vi "Shortcut Menu from Cluster.vi"() -> ()   [LabVIEW 2019]
doc: "An example of using a cluster of enums and booleans to provide menu options, both for the right-click menu of a control, and in the VI menu bar."
uses:
  vi.lib/JDP Science/JDP Science Common Utilities/Shortcut Menu Tools/Menu From Cluster.lvlib
panel:
  out "Item":string
  out "ItemTag":string
  out "A control":dbl caption="Run this program, then right-click this control and experiment changing Options"
  # "This example also shows how to add the same Options to the VI's menu bar (under \"User Options\")."
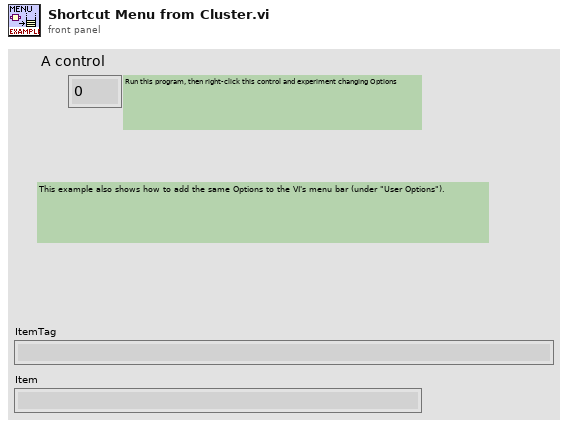
[diagram p1: front panel]
types:
  T1 = cluster{"An Enum":enum16{"Item1", "Item2", "Item3"}, "A Boolean":bool, "Another boolean":bool, "A subcluster":cluster{"Sub Enum":enum16{"Item1", "Item2", "Item3"}, "Sub Boolean":bool, "Subsubcluster":cluster{"Sub Sub Enum":enum16{"Item1", "Item2", "Item3"}, "Sub Sub Boolean":bool, "3sub":cluster{"3sub Enum":enum16{"Item1", "Item2", "Item3"}, "3sub Boolean":bool}}}}
  T2 = cluster{"Options Menu":cluster{"An Enum":enum16{"Item1", "Item2", "Item3"}, "A Boolean":bool, "Another boolean":bool, "A subcluster":cluster{"Sub Enum":enum16{"Item1", "Item2", "Item3"}, "Sub Boolean":bool, "Subsubcluster":cluster{"Sub Sub Enum":enum16{"Item1", "Item2", "Item3"}, "Sub Sub Boolean":bool, "3sub":cluster{"3sub Enum":enum16{"Item1", "Item2", "Item3"}, "3sub Boolean":bool}}}}}
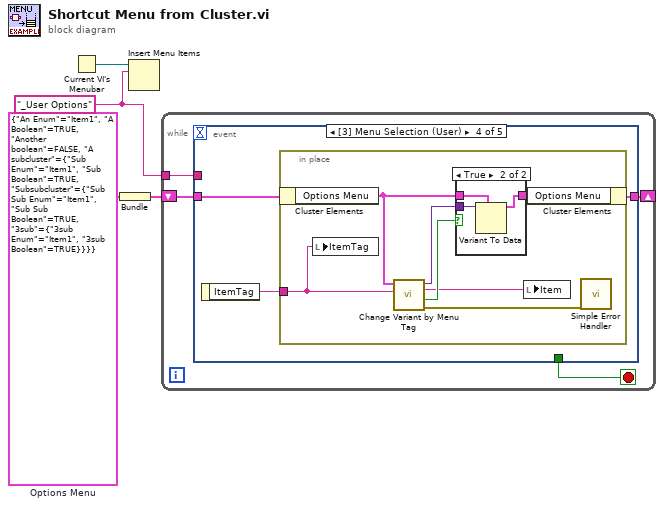
[diagram p0: block diagram]
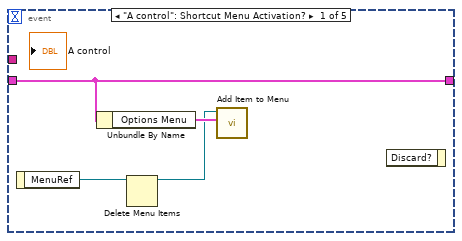
[diagram p2: hidden frame]
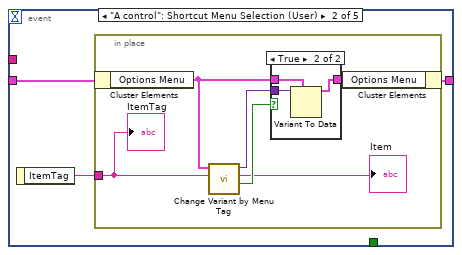
[diagram p3: hidden frame]
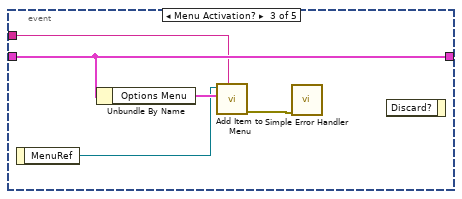
[diagram p5: hidden frame]
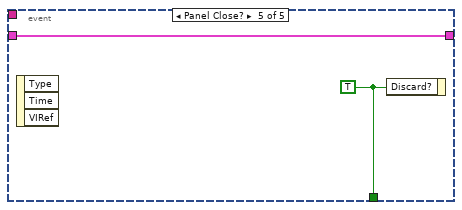
[diagram p7: hidden frame]
diagram:
  w1 = "_User Options" ("menu tag")
  w3 = T1 {"An Enum"=enum."Item1", "A Boolean"=TRUE, "Another boolean"=FALSE, "A subcluster"={"Sub Enum"=enum."Item1", "Sub Boolean"=TRUE, "Subsubcluster"={"Sub Sub Enum"=enum."Item1", "Sub Sub Boolean"=TRUE, "3sub"={"3sub Enum"=enum."Item1", "3sub Boolean"=TRUE}}}}  # Options Menu
  n1 = Current VI's Menubar() -> (w2:refnum<k9>)
  n2 = Bundle("Options Menu"=w3) -> (w4:T2)  [unwired: 1 in]
  n3 = Insert Menu Items(8:w1, 9:w2) -> ()  [unwired: 4 in, 3 out]
  n4 = while {
    shift-right: [w7] -> _
    shift-left: w4 -> [w8]
    tunnel: w1 -> [w5]
    stop <- w6 stop-if-true
    n5 = event shown="[3] Menu Selection (User)" {
      selector: _ -> [_ _ _ _ _]
      dyn-events: _ -> [_ _ _ _ _]
      timeout: _ -> [_ _ _ _ _]
      tunnel: w8 -> [w12 w15 w30 w33 w46]
      tunnel: [w12 w14 w30 w32 w46] -> w7
      tunnel: [_ _ _ _ w45] -> w6
      tunnel: w5 -> [_ _ w28 _ _]
      event "A control": Shortcut Menu Activation? {
        n6 = event-data() -> ("MenuRef"=w11:refnum<k9>)  [unwired: 1 in]
        n7 = Unbundle By Name(w12) -> ("Options Menu"=w10:T1)
        n8 = Delete Menu Items(9:w11) -> (3:w9:refnum<k9>)  [unwired: 3 in, 1 out]
        n9 = call "Add Item to Menu.vi"("Item(s) to Add"=w10, "menu reference"=w9) -> ()  [unwired: 7 in, 3 out]
        n10 = event-data() -> ()  [unwired: 2 in, 1 out]
      }
      event "A control": Shortcut Menu Selection (User) {
        n11 = event-data() -> ("ItemTag"=w13:string)  [unwired: 1 in]
        n12 = in-place {
          in-place-border: w13 -> [w17]
          n13 = in-place-cluster #1(w15) -> ("Options Menu"=w20:T1)
          n14 = call "Change Variant by Menu Tag.vi"("tag"=w17, "Cluster"=w20) -> ("Cluster Changed"=w18:bool, "Item"=→"Item":string, "VCluster out"=w19:variant)  [unwired: 6 in, 1 out]
          n15 = case shown="True" w18 {
            tunnel: w19 -> [_ w25]
            tunnel: [w22 w24] -> w21
            tunnel: w20 -> [w22 w23]
            frame False {
            }
            frame True {
              n16 = Variant To Data(type=w23, Variant=w25) -> (data=w24:T1)  [unwired: 1 in, 1 out]
            }
          }
          n17 = in-place-cluster #1("Options Menu"=w21) -> (w14:T2)
          "ItemTag" <- w17
        }
      }
      event Menu Activation? {
        n18 = event-data() -> ("MenuRef"=w27:refnum<k9>)  [unwired: 1 in]
        n19 = Unbundle By Name(w30) -> ("Options Menu"=w29:T1)
        n20 = call "Add Item to Menu.vi"("menu tag"=w28, "Item(s) to Add"=w29, "menu reference"=w27) -> ("error out"=w26:errorcluster)  [unwired: 6 in, 2 out]
        n21 = call <vilib>:"Simple Error Handler.vi"("error in (no error)"=w26) -> ()  [unwired: 4 in, 5 out]
        n22 = event-data() -> ()  [unwired: 2 in, 1 out]
      }
      event Menu Selection (User) {
        n23 = event-data() -> ("ItemTag"=w31:string)  [unwired: 1 in]
        n24 = in-place {
          in-place-border: w31 -> [w36]
          n25 = in-place-cluster #2(w33) -> ("Options Menu"=w39:T1)
          n26 = local write "ItemTag"(w36) -> ()
          n27 = call "Change Variant by Menu Tag.vi"("tag"=w36, "Cluster"=w39) -> ("error out"=w34:errorcluster, "Cluster Changed"=w37:bool, "Item"=w35:string, "VCluster out"=w38:variant)  [unwired: 6 in]
          n28 = case shown="True" w37 {
            tunnel: w38 -> [_ w44]
            tunnel: [w41 w43] -> w40
            tunnel: w39 -> [w41 w42]
            frame False {
            }
            frame True {
              n29 = Variant To Data(type=w42, Variant=w44) -> (data=w43:T1)  [unwired: 1 in, 1 out]
            }
          }
          n30 = local write "Item"(w35) -> ()
          n31 = in-place-cluster #2("Options Menu"=w40) -> (w32:T2)
          n32 = call <vilib>:"Simple Error Handler.vi"("error in (no error)"=w34) -> ()  [unwired: 4 in, 5 out]
        }
      }
      event Panel Close? {
        w45 = TRUE
        n33 = event-data() -> ()  [unwired: 1 in, 3 out]
        n34 = event-data("Discard?"=w45) -> ()  [unwired: 1 in, 1 out]
      }
    }
  }
